vi "res.vi"() -> ()   [LabVIEW 2016]
uses:
  <vilib>/UPVI/lvhdf5/file.llb/LVH5F Operation.ctl
  <vilib>/UPVI/lvhdf5/dataset.llb/LVH5D Operation.ctl
  <vilib>/Utility/miscctls.llb/LVRectTypeDef.ctl
  <vilib>/UPVI/lvhdf5/group.llb/H5G_obj_t.ctl
  <vilib>/functionblocks/Accumulate/Collect Numeric Array/Collect Numeric Array.vi
  <vilib>/UPVI/lvhdf5/utility.llb/Select HDF5 Dialog.vi
  <vilib>/UPVI/lvhdf5/utility.llb/Select HDF5 Dialog (Object Only).vi
  <vilib>/UPVI/lvhdf5/dataset.llb/Simple H5Dwrite (Variant).vi
  <vilib>/functionblocks/FB Core/FB Core.xnode
  <vilib>/UPVI/lvhdf5/dataset.llb/Simple H5Dwrite.xnode
  <vilib>/UPVI/lvhdf5/library.llb/HDF5 Ref.ctl
  <instrlib>/Ocean Optics 2000 4000/Ocean Optics 2000 4000.lvlib
  <vilib>/functionblocks/NI_FunctionBlock Libraries.lvlib
  <vilib>/UPVI/lvhdf5/identifier.llb/Not an HDF5 Refnum Constant.vi
  <vilib>/Utility/error.llb/Error Cluster From Error Code.vi
  <vilib>/UPVI/lvhdf5/dataset.llb/OpenCreateReplace Dataset by Element Type.vi
  <vilib>/UPVI/lvhdf5/dataspace.llb/H5Sselect_hyperslab.vi
  <vilib>/UPVI/lvhdf5/dataset.llb/H5Dwrite (Variant).vi
  <vilib>/UPVI/lvhdf5/dataset.llb/H5Dget_space.vi
  <vilib>/UPVI/lvhdf5/attribute.llb/private/LVH5AwriteWDTAttrs.vi
  <vilib>/UPVI/lvhdf5/dataspace.llb/H5Sclose.vi
  <vilib>/UPVI/lvhdf5/dataset.llb/H5Dclose.vi
  <vilib>/UPVI/lvhdf5/utility.llb/Select HDF5 Dialog (File and Object).vi
panel:
  in  "Enable Strobe (Disabled)":bool
  out "Spectral Waveform":cluster{dbl[], dbl[]}(graph)
  in  "Ruta":path=path "C:/Users/Posgrado/Desktop/Test/Prueba"
  in  "Dataset Path":string
  out "Longitud de onda":dbl[](array[numeric])
  out "Espectro":dbl[](array[numeric])
  out "full":bool
  out "points collected":i32=10
  in  "Reset":bool
  in  "Guarda muestra":bool
  in  "No. de muestras":u32=1
  out "Wavelength (nm)":dbl[](array[numeric])
  out "Spectrum by Pixel Number":dbl[](array[numeric])
  in  "VISA resource name":refnum<visa-resource-name>="USB0::0x2457::0x1012::NI-VISA-10002::RAW"
  in  "stop":bool
  out "Guarda datos":bool
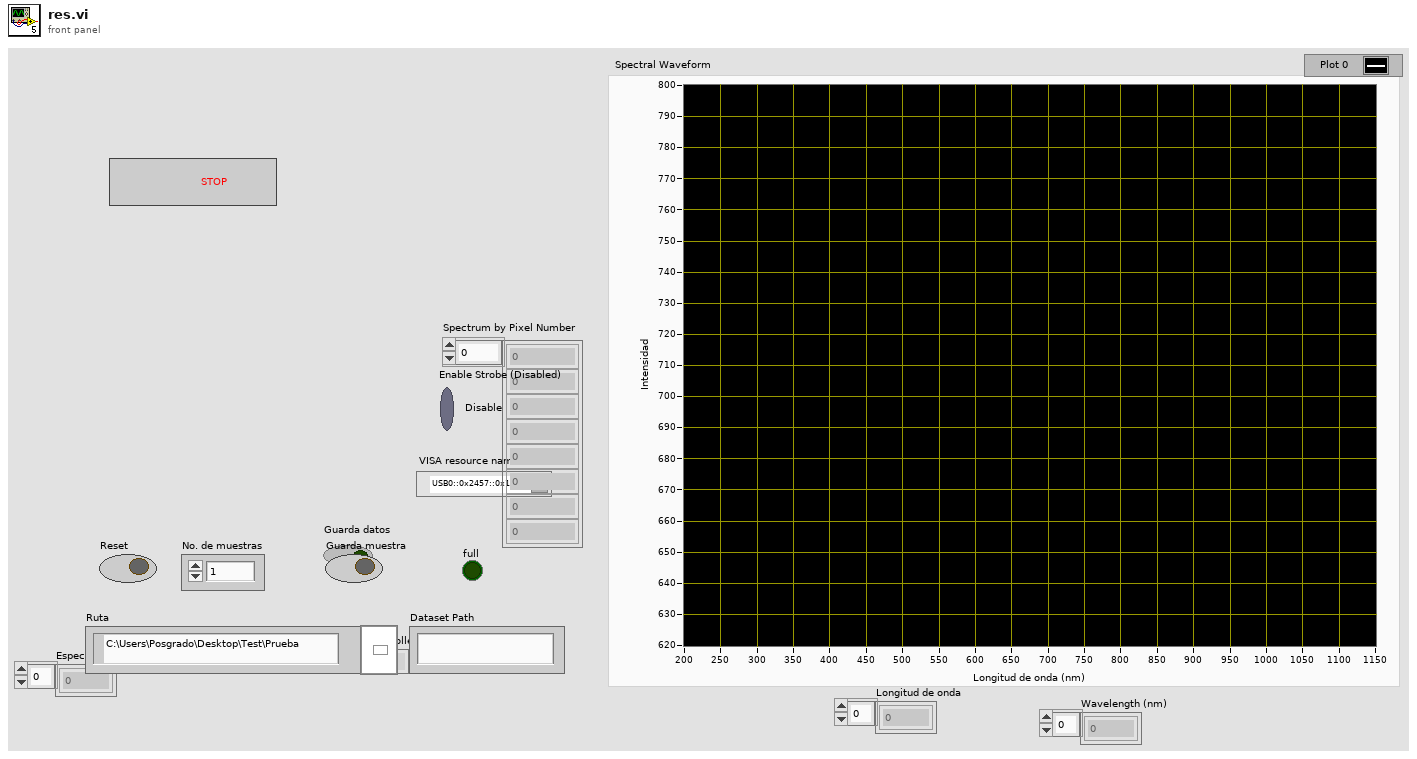
[diagram p1: front panel]
types:
  T1 = typedef "LVH5D Operation.ctl" = enum16{"open", "replace", "create", "open or create", "create or replace", "create or replace with confirmation"}
  T2 = typedef "LVH5F Operation.ctl" = enum16{"open", "open or create", "create or replace", "create or replace (with confirmation)", "create", "open (read only)"}
  T3 = typedef "LVRectTypeDef.ctl" = cluster{"Left":i16, "Top":i16, "Right":i16, "Bottom":i16}
  T4 = cluster{"Behavior":enum32{"Invalid", "Default", "Floating", "Floating/Auto-Hide", "Modal"}, "Position":T3, "Center":bool, "Title":string}
  T5 = typedef "H5G_obj_t.ctl" = i32
  T6 = cluster{"Object Types (any)":T5[], "Object Pattern":string}
  T7 = typedef "HDF5 Ref.ctl" = refnum<k1>
  T8 = cluster{"Wavelength (nm)":dbl[], "Spectrum by Pixel Number":dbl[]}
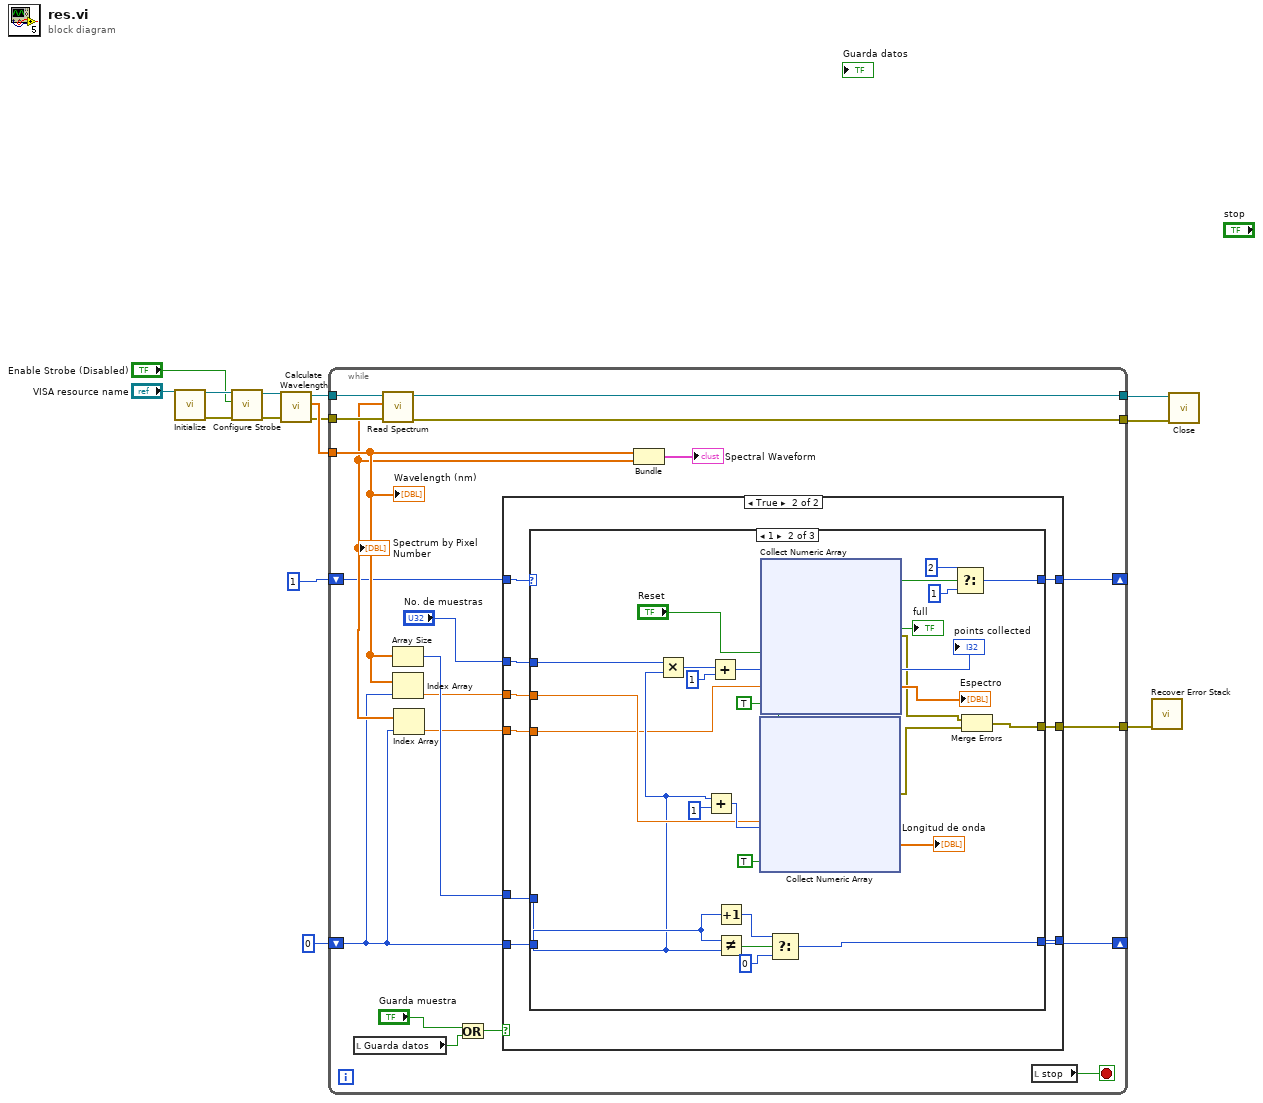
[diagram p0: block diagram]
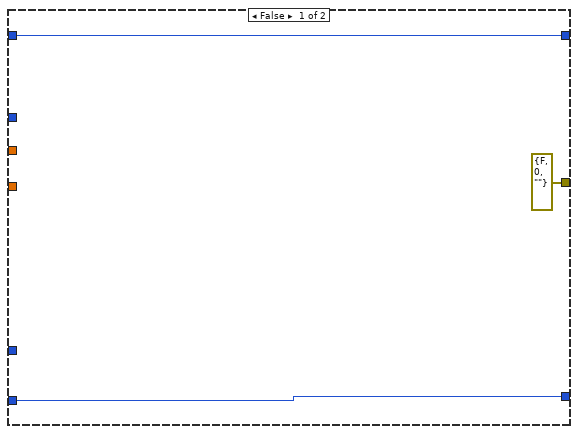
[diagram p2: hidden frame]
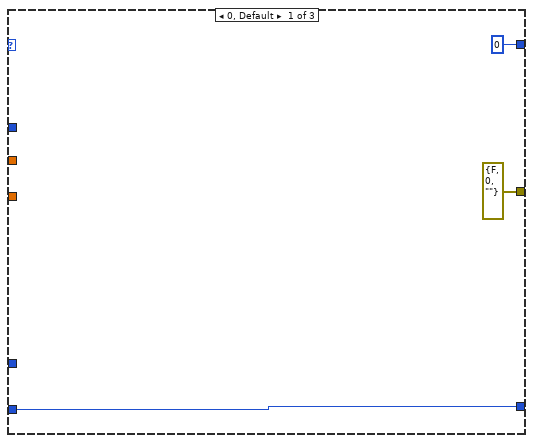
[diagram p3: hidden frame]
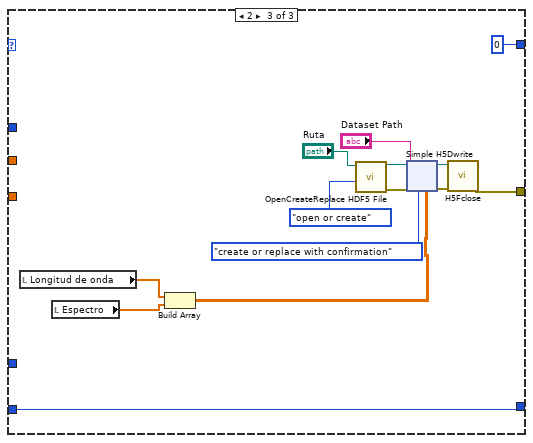
[diagram p4: hidden frame]
diagram:
  n1 = call <instrlib>:"Initialize.vi"("VISA resource name"="VISA resource name") -> ("error out"=w13:errorcluster, "VISA resource name out"=w14:refnum<visa-resource-name>)  [unwired: 2 in, 7 out]
  n2 = call <instrlib>:"Configure Strobe.vi"("error in (no error)"=w13, "Enable Strobe (Disabled)"="Enable Strobe (Disabled)", "VISA resource name"=w14) -> ("error out"=w4:errorcluster, "VISA resource name out"=w5:refnum<visa-resource-name>)  [unwired: 7 out]
  n3 = call <instrlib>:"Calculate Wavelength.vi"("error in (no error)"=w4, "VISA resource name"=w5) -> ("error out"=w6:errorcluster, "Wavelength (nm)"=w8:dbl[], "VISA resource name out"=w7:refnum<visa-resource-name>)  [unwired: 1 in, 6 out]
  n4 = while {
    tunnel: [w34] -> w11
    tunnel: [w33] -> w10
    tunnel: w8 -> [w29]
    tunnel: w7 -> [w32]
    tunnel: w6 -> [w31]
    shift-right: [w27] -> _
    shift-left: 0 -> [w25]
    shift-right: [w21] -> _
    shift-left: 1 -> [w22]
    tunnel: [w19] -> w1
    stop <- w18 stop-if-true
    n5 = local read "Guarda datos"() -> (w15:bool)
    n6 = call <instrlib>:"Read Spectrum.vi"("error in (no error)"=w31, "VISA resource name"=w32) -> ("error out"=w33:errorcluster, "Spectrum by Pixel Number"=w28:dbl[], "VISA resource name out"=w34:refnum<visa-resource-name>)  [unwired: 6 in, 1 out]
    "Spectrum by Pixel Number" <- w28
    n7 = Array Size(array=w29) -> (size(s)=w26:i32)
    n8 = Index Array(array=w29, index=w25) -> (element=w24:dbl)
    n9 = Index Array(array=w28, index=w25) -> (element=w20:dbl)
    n10 = Or(x="Guarda muestra", y=w15) -> (x .or. y?=w17:bool)
    n11 = case shown="True" w17 {
      tunnel: w25 -> [w37 w45]
      tunnel: [w37 w46] -> w27
      tunnel: w26 -> [_ w44]
      tunnel: w24 -> [_ w43]
      tunnel: "No. de muestras" -> [_ w42]
      tunnel: w22 -> [w36 w41]
      tunnel: [w36 w40] -> w21
      tunnel: w20 -> [_ w39]
      tunnel: [errorcluster {"status"=FALSE, "code"=0, "source"=""} ("error out") w38] -> w19
      frame False {
      }
      frame True {
        n12 = case shown="1" w41 {
          tunnel: [w49 w75 w190] -> w46
          tunnel: w45 -> [w49 w72 w190]
          tunnel: w44 -> [_ w63 _]
          tunnel: w43 -> [_ w69 _]
          tunnel: w42 -> [_ w67 _]
          tunnel: [0 w58 0] -> w40
          tunnel: w39 -> [_ w60 _]
          tunnel: [errorcluster {"status"=FALSE, "code"=0, "source"=""} ("error out") w52 w189] -> w38
          frame 0, Default {
          }
          frame 1 {
            n13 = Multiply(x=w67, y=w63) -> (x*y=w66:u32)
            n14 = Add(x=w63, y=1) -> (x+y=w71:i32)
            n15 = Add(x=w66, y=u32 1) -> (x+y=w64:u32)
            n16 = Increment(x=w72) -> (x+1=w76:i32)
            n17 = Not Equal?(x=w72, y=w63) -> (x != y?=w73:bool)
            n18 = xnode "Collect Numeric Array"("reset"="Reset", "array size"=w71, "input"=w69, "enable"=TRUE) -> ("error out"=w53:errorcluster, "collected data"=→"Longitud de onda":dbl[])  [unwired: 1 in, 2 out]
            n19 = xnode "Collect Numeric Array"("reset"="Reset", "array size"=w64, "input"=w60, "enable"=TRUE) -> ("error out"=w51:errorcluster, "full"=w57:bool, "points collected"=→"points collected":i32, "collected data"=→"Espectro":dbl[])  [unwired: 1 in]
            "full" <- w57
            n20 = Select(t=w76, s=w73, f=0) -> (s? t:f=w75:i32)
            n21 = Select(t=2, s=w57, f=1) -> (s? t:f=w58:i32)
            n22 = Merge Errors(w51, w53) -> (w52:errorcluster)
          }
          frame 2 {
            n23 = local read "Longitud de onda"() -> (w177:dbl[])
            n24 = local read "Espectro"() -> (w178:dbl[])
            n25 = Build Array(w177, w178) -> (w179:dbl[][])
            n26 = call <vilib>:"OpenCreateReplace HDF5 File.vi"("function (open or create)"=LVH5F_Operation."open or create", "path"="Ruta") -> ("error out"=w185:errorcluster, "HDF5 Ref out"=w184:T7)  [unwired: 6 in]
            n27 = xnode "Simple H5Dwrite"("Dataset Path"="Dataset Path", "error in (no error)"=w185, "operation (open or create)"=LVH5D_Operation."create or replace with confirmation", "HDF5 Path or Ref"=w184, "Data"=w179) -> ("HDF5 Ref out"=w181:T7, "error out"=w182:errorcluster)  [unwired: 3 in, 1 out]
            n28 = call <vilib>:"H5Fclose.vi"("error in (no error)"=w182, "HDF5 Ref"=w181) -> ("error out"=w189:errorcluster)  [unwired: 7 in]
          }
        }
      }
    }
    n29 = Bundle("Wavelength (nm)"=w29, "Spectrum by Pixel Number"=w28) -> (→"Spectral Waveform":T8)  [unwired: 1 out]
    n30 = local read "stop"() -> (w18:bool)
    "Wavelength (nm)" <- w29
  }
  n31 = call <vilib>:"Recover Error Stack.vi"("error in (no error)"=w1) -> ()  [unwired: 5 in, 4 out]
  n32 = call <instrlib>:"Close.vi"("error in (no error)"=w10, "VISA resource name"=w11) -> ()  [unwired: 10 out]
